vi "Read CtlRef.vi"(8 "error in (no error)":errorcluster, 11 "TreeDoubleClickMsg in":refnum<class "TreeDoubleClickMsg.lvclass">) -> (0 "error out":errorcluster, 2 "CtlRef":refnum<vi>, 3 "TreeDoubleClickMsg out":refnum<class "TreeDoubleClickMsg.lvclass">)   [LabVIEW 2017, in "ActorEvents.lvlib" / "TreeDoubleClickMsg.lvclass"]
uses:
  TreeDoubleClickMsg.lvclass
  TreeDoubleClickMsg.lvclass/TreeDoubleClickMsg.ctl
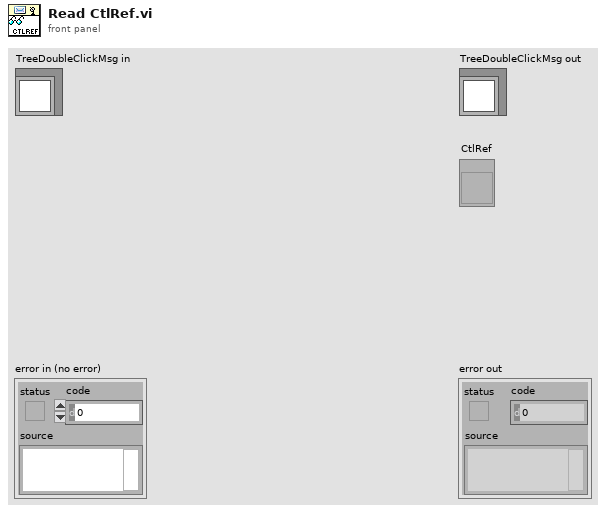
[diagram p1: front panel]
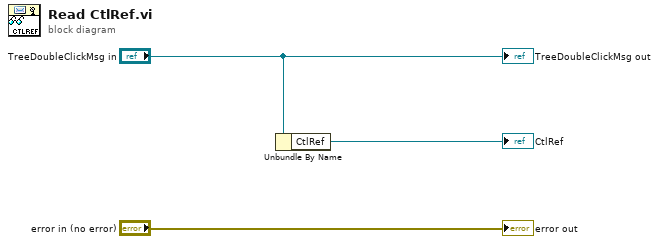
[diagram p0: block diagram]
diagram:
  n1 = Unbundle By Name("TreeDoubleClickMsg in") -> ("CtlRef"=→"CtlRef":refnum<vi>)
  "error out" <- "error in (no error)"
  "TreeDoubleClickMsg out" <- "TreeDoubleClickMsg in"
